vi "Get UUID.vi"(8 "error in (no error)":errorcluster, 11 "output_actor in":refnum<class "Output Actor.lvclass">) -> (0 "error out":errorcluster, 2 "UUID":string, 3 "output_actor out":refnum<class "Output Actor.lvclass">)   [LabVIEW 2015, in "Output Actor.lvclass"]
uses:
  Output Actor.lvclass
  Output Actor.lvclass/Output Actor.ctl
  output/Output.lvclass
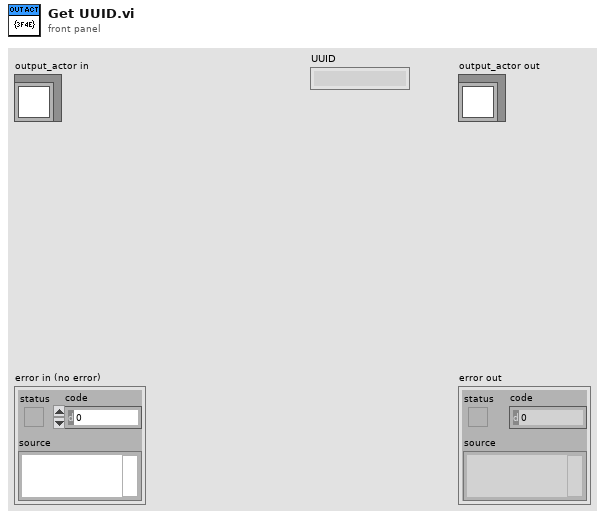
[diagram p1: front panel]
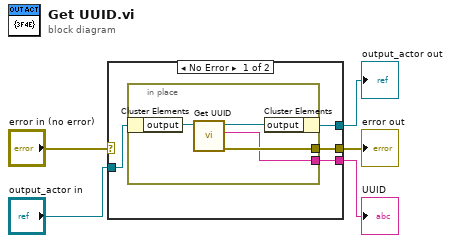
[diagram p0: block diagram]
diagram:
  n1 = case shown="No Error" "error in (no error)" {
    selector: "error in (no error)" -> [_ w15]
    tunnel: [w7 w15] -> w4
    tunnel: [w8 w14] -> w2
    tunnel: "output_actor in" -> [w9 w14]
    tunnel: [w6 _] -> w1
    frame No Error {
      n2 = in-place {
        in-place-border: [w11] -> w7
        in-place-border: [w10] -> w6
        n3 = in-place-cluster #1(w9) -> ("output"=w13:refnum<class "Output.lvclass">)
        n4 = call "Get UUID.vi"("Output in"=w13) -> ("error out"=w11:errorcluster, "UUID"=w10:string, "Output out"=w12:refnum<class "Output.lvclass">)  [unwired: 8 in]
        n5 = in-place-cluster #1("output"=w12) -> (w8:refnum<class "Output Actor.lvclass">)
      }
    }
    frame Error {
    }
  }
  "error out" <- w4
  "output_actor out" <- w2
  "UUID" <- w1
